vi "Setting[].vi"(8 "error in (no error)":errorcluster, 11 "Save Restore Settings in":refnum<class "Save Restore Settings.lvclass">) -> (0 "error out":errorcluster, 1 "Value[]":variant[](array[variant]), 2 "Tag[]":string[](array[string]), 3 "Save Restore Settings out":refnum<class "Save Restore Settings.lvclass">)   [LabVIEW 2020, in "Save Restore Settings.lvclass"]
uses:
  <userlib>/_MGI/Application Control/MGI Save Restore Settings/Save Restore Settings.lvclass
  <userlib>/_MGI/Application Control/MGI Save Restore Settings/Save Restore Settings.lvclass/Save Restore Settings.ctl
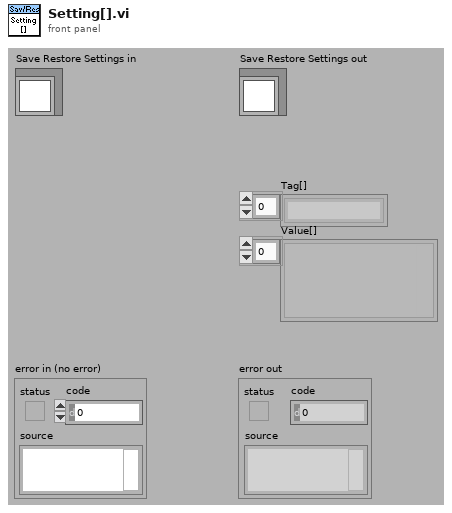
[diagram p1: front panel]
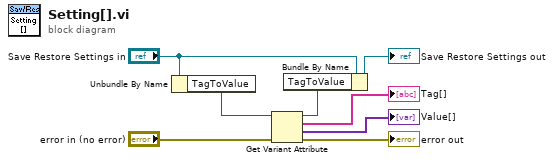
[diagram p0: block diagram]
diagram:
  n1 = Unbundle By Name("Save Restore Settings in") -> ("TagToValue"=w6:variant)
  n2 = Get Variant Attribute(Variant=w6, error in="error in (no error)") -> (duplicate Variant=w3:variant, names=→"Tag[]":string[], values=→"Value[]":variant[], error out=→"error out":errorcluster)  [unwired: 2 in]
  n3 = Bundle By Name(cluster="Save Restore Settings in", "TagToValue"=w3) -> (→"Save Restore Settings out":refnum<class "Save Restore Settings.lvclass">)
